vi "Get Functions Path.vi"(11 "error in":errorcluster) -> (4 "Basic Function List":path, 6 "Instrument IO":path, 15 "error out":errorcluster)   [LabVIEW 2019, in "LSL.lvlib" / "scripts manager.lvclass"]
uses:
  scripts manager.lvclass
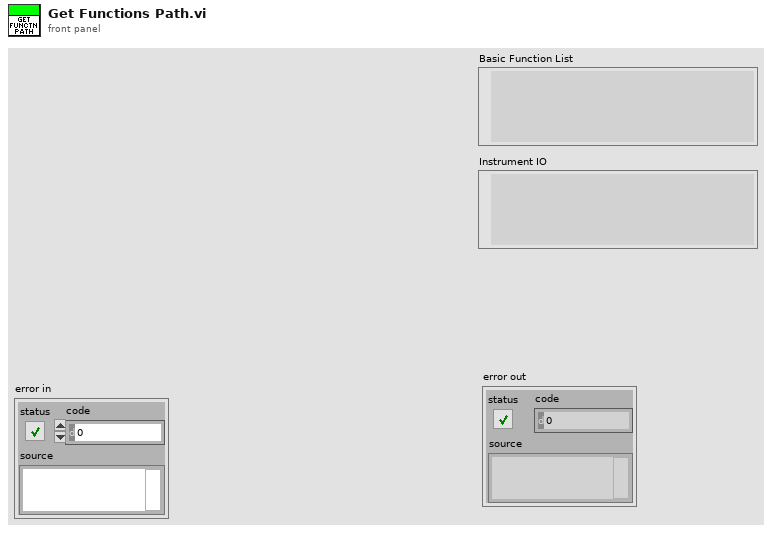
[diagram p1: front panel]
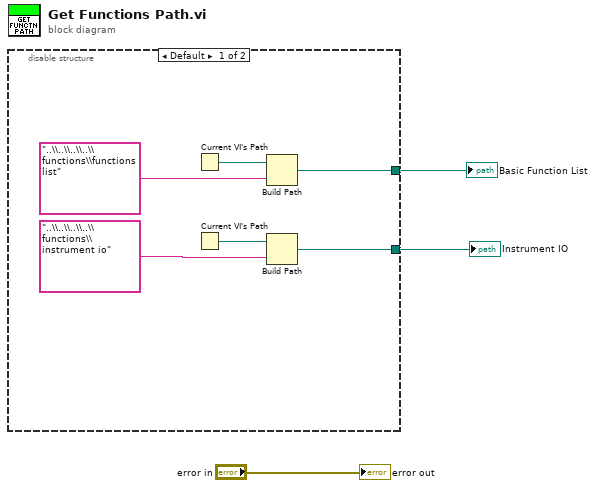
[diagram p0: block diagram]
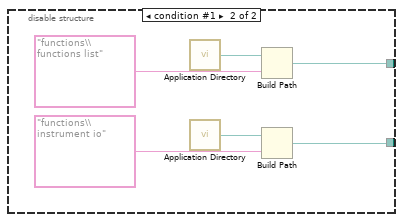
[diagram p2: hidden frame]
diagram:
  n1 = disable-structure shown="Default" {
    disable-tunnel: [w8 w14] -> w2
    disable-tunnel: [w4 w10] -> w1
    frame condition #0 (active) {
      n2 = Current VI's Path() -> (path=w7:path)
      n3 = Current VI's Path() -> (path=w6:path)
      n4 = Build Path(base path=w7, name or relative path="..\\..\\..\\..\\functions\\functions list") -> (appended path=w8:path)
      n5 = Build Path(base path=w6, name or relative path="..\\..\\..\\..\\functions\\instrument io") -> (appended path=w4:path)
    }
    frame condition #1 {
      n6 = call <vilib>:"Application Directory.vi"() -> ("Application Directory"=w13:path)
      n7 = call <vilib>:"Application Directory.vi"() -> ("Application Directory"=w12:path)
      n8 = Build Path(base path=w13, name or relative path="functions\\functions list") -> (appended path=w14:path)
      n9 = Build Path(base path=w12, name or relative path="functions\\instrument io") -> (appended path=w10:path)
    }
  }
  "Basic Function List" <- w2
  "Instrument IO" <- w1
  "error out" <- "error in"
